vi "CRYStd header parse.vi"(10 "Main info cluster":T2, 11 "x-y settings array":T1 {"yp db ref" format="%.2f"; "ym db ref" format="%.2f"; "x db ref" format="%.2f"}) -> (3 "x-y settings array out":T1 {"yp db ref" format="%.2f"; "ym db ref" format="%.2f"; "x db ref" format="%.2f"})   [LabVIEW 2013]
uses:
  Control/CRYImp wiz main info.ctl
  Control/CRYx-y settings array.ctl
  CRYImp wiz global.vi
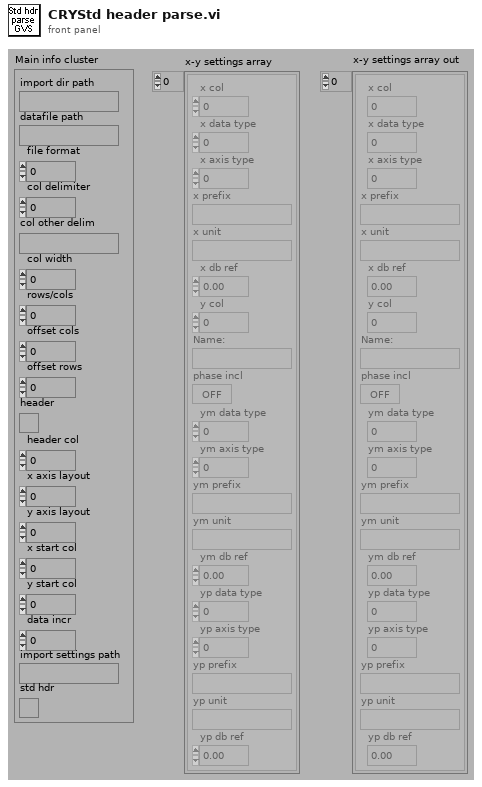
[diagram p1: front panel]
types:
  T1 = typedef "CRYx-y settings array.ctl" = cluster{"x col":i32, "x data type":u16, "x axis type":u16, "x prefix":string, "x unit":string, "x db ref":dbl, "y col":i32, "Name:":string, "phase incl":bool, "ym data type":u16, "ym axis type":u16, "ym prefix":string, "ym unit":string, "ym db ref":dbl, "yp data type":u16, "yp axis type":u16, "yp prefix":string, "yp unit":string, "yp db ref":dbl}[]
  T2 = typedef "CRYImp wiz main info.ctl" = cluster{"import dir path":path, "datafile path":path, "file format":i32, "col delimiter":i32, "col other delim":string, "col width":i32, "rows/cols":i32, "offset cols":i32, "offset rows":i32, "header":bool, "header col":i32, "x axis layout":i32, "y axis layout":i32, "x start col":i32, "y start col":i32, "data incr":i32, "import settings path":path, "std hdr":bool}
  T3 = cluster{"x col":i32, "x data type":u16, "x axis type":u16, "x prefix":string, "x unit":string, "x db ref":dbl, "y col":i32, "Name:":string, "phase incl":bool, "ym data type":u16, "ym axis type":u16, "ym prefix":string, "ym unit":string, "ym db ref":dbl, "yp data type":u16, "yp axis type":u16, "yp prefix":string, "yp unit":string, "yp db ref":dbl}
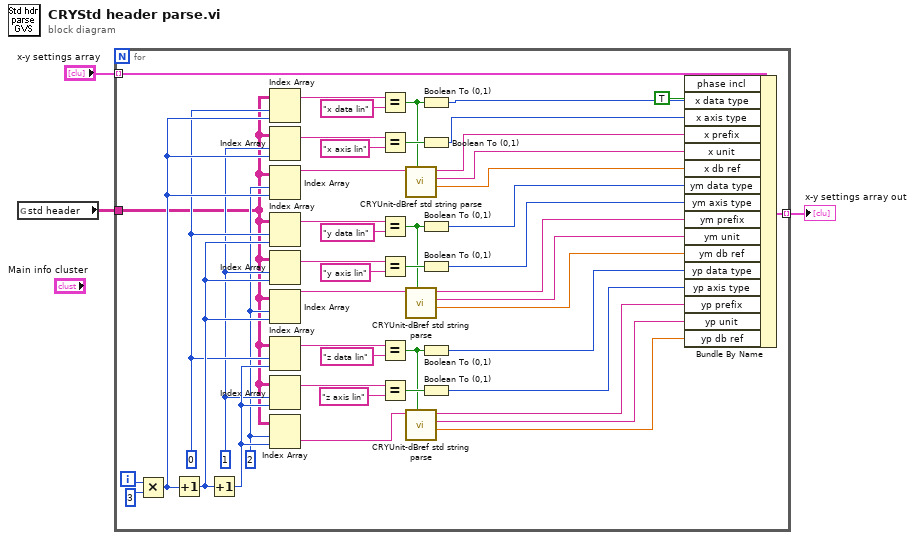
[diagram p0: block diagram]
diagram:
  n1 = global read "CRYImp wiz global.vi" "std header"() -> (w2:string[][])
  n2 = for {
    tunnel: "x-y settings array" -> [w50] mode=indexing
    tunnel: w2 -> [w41]
    tunnel: [w4] -> w1 mode=indexing
    i -> [w48]
    w42 = 2
    w43 = 1
    w44 = 0
    n3 = Multiply(x=w48, y=3) -> (x*y=w47:i32)
    n4 = Increment(x=w47) -> (x+1=w46:i32)
    n5 = Increment(x=w46) -> (x+1=w45:i32)
    n6 = Index Array(array=w41, index (row)=w44, index (col)=w47) -> (element=w39:string)
    n7 = Index Array(array=w41, index (row)=w43, index (col)=w47) -> (element=w36:string)
    n8 = Index Array(array=w41, index (row)=w42, index (col)=w47) -> (element=w19:string)
    n9 = Index Array(array=w41, index (row)=w44, index (col)=w46) -> (element=w29:string)
    n10 = Index Array(array=w41, index (row)=w43, index (col)=w46) -> (element=w28:string)
    n11 = Index Array(array=w41, index (row)=w42, index (col)=w46) -> (element=w18:string)
    n12 = Index Array(array=w41, index (row)=w44, index (col)=w45) -> (element=w27:string)
    n13 = Index Array(array=w41, index (row)=w43, index (col)=w45) -> (element=w26:string)
    n14 = Index Array(array=w41, index (row)=w42, index (col)=w45) -> (element=w17:string)
    n15 = Equal?(x=w39, y="x data lin") -> (x = y?=w7:bool)
    n16 = Equal?(x=w36, y="x axis lin") -> (x = y?=w37:bool)
    n17 = Equal?(x=w29, y="y data lin") -> (x = y?=w6:bool)
    n18 = Equal?(x=w28, y="y axis lin") -> (x = y?=w33:bool)
    n19 = Equal?(x=w27, y="z data lin") -> (x = y?=w5:bool)
    n20 = Equal?(x=w26, y="z axis lin") -> (x = y?=w30:bool)
    n21 = call "CRYUnit-dBref std string parse.vi"("Linear data"=w7, "Std. header string in"=w19) -> ("dB ref"=w14:dbl, "Unit"=w15:string, "Prefix"=w16:string)  [unwired: 7 in]
    n22 = call "CRYUnit-dBref std string parse.vi"("Linear data"=w6, "Std. header string in"=w18) -> ("dB ref"=w11:dbl, "Unit"=w12:string, "Prefix"=w13:string)  [unwired: 7 in]
    n23 = call "CRYUnit-dBref std string parse.vi"("Linear data"=w5, "Std. header string in"=w17) -> ("dB ref"=w8:dbl, "Unit"=w9:string, "Prefix"=w10:string)  [unwired: 7 in]
    n24 = Boolean To (0,1)(Boolean=w7) -> (0, 1=w38:i16)
    n25 = Boolean To (0,1)(Boolean=w37) -> (0, 1=w35:i16)
    n26 = Boolean To (0,1)(Boolean=w6) -> (0, 1=w23:i16)
    n27 = Boolean To (0,1)(Boolean=w33) -> (0, 1=w22:i16)
    n28 = Boolean To (0,1)(Boolean=w5) -> (0, 1=w21:i16)
    n29 = Boolean To (0,1)(Boolean=w30) -> (0, 1=w20:i16)
    n30 = Bundle By Name(cluster=w50, "phase incl"=TRUE ("Bundle Element"), "x data type"=w38, "x axis type"=w35, "x prefix"=w16, "x unit"=w15, "x db ref"=w14, "ym data type"=w23, "ym axis type"=w22, "ym prefix"=w13, "ym unit"=w12, "ym db ref"=w11, "yp data type"=w21, "yp axis type"=w20, "yp prefix"=w10, "yp unit"=w9, "yp db ref"=w8) -> (w4:T3)
  }
  "x-y settings array out" <- w1
